vi "ModbusTestHmi.vi"() -> ()   [LabVIEW 2018, in "ModbusTestMasterLibrary.lvlib"]
uses:
  ModbusTestMasterLibrary.lvlib
panel:
  out "Cycle":i32
  in  "stop":bool
  out "Input Registry #2 (30002)":u16(slide) scale=0.0..1024.0
  in  "Holding Registry #2 (40002)":u16(slide) scale=0.0..255.0
  in  "Holding Registry #1 (40001)":u16(slide) scale=0.0..255.0
  in  "Coil #2 (00002)":bool
  in  "Coil #1 (00001)":bool
  out "Input Registry #1 (30001)":u16(slide) scale=0.0..1024.0
  out "Discrete Input #2 (10002)":bool
  out "Discrete Input #1 (10001)":bool
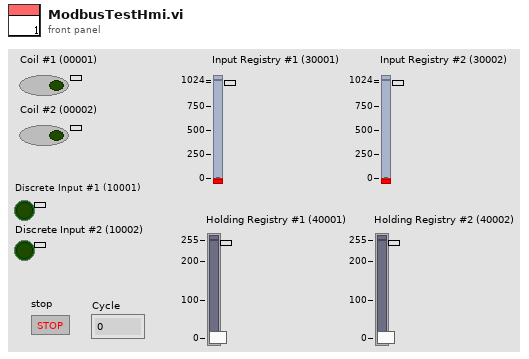
[diagram p1: front panel]
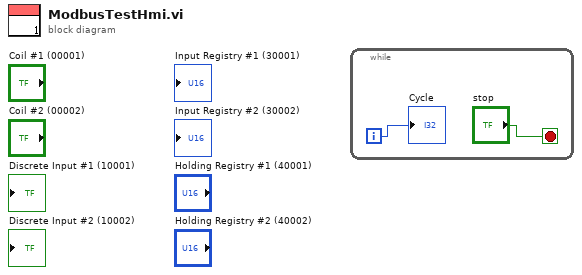
[diagram p0: block diagram]
diagram:
  n1 = while {
    i -> [w2]
    stop <- "stop" stop-if-true
    "Cycle" <- w2
  }
